vi "modify channel test.vi"() -> ()   [LabVIEW 2013, in "TEC tests.lvlib"]
uses:
  TEC tests.lvlib
  <vilib>/NI/Tag Bus Module Framework/channel/channel classification.ctl
  configuration/TEC configuration.lvclass
  configuration/TEC configuration.lvclass/TEC configuration.ctl
  <vilib>/NI/Tag Bus Module Framework/channel/TBM channel.lvclass/TBM channel.ctl
  <vilib>/NI/Tag Bus/tag/tag descriptor.lvclass/tag descriptor.ctl
  <vilib>/NI/Tag Bus Module Framework/channel/Read channel classification.vi
  <vilib>/NI/Tag Bus Module Framework/channel/Write channel classification.vi
  <vilib>/NI/Tag Bus/tag/read tag name.vi
  configuration/Write channels.vi
  <vilib>/NI/Tag Bus Module Framework/channel/TBM channel.lvclass
  <vilib>/NI/Tag Bus Module Framework/root configuration/TBM configuration.lvclass
panel:
  out "rename success":bool
  out "no err":errorcluster
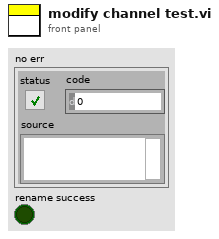
[diagram p1: front panel]
types:
  T1 = typedef "TBM channel.lvclass/channel classification.ctl" = enum16{"input data", "output data", "processing parameter", "processing result"}
  T2 = typedef "tag bus.lvlib/tag descriptor.lvclass/Data Type.ctl" = enum16{"Double", "Single", "I64", "I32", "I16", "I8", "U64", "U32", "U16", "U8", "Boolean", "String", "Array of Double", "Array of Single", "Array of I64", "Array of I32", "Array of I16", "Array of I8", "Array of U64", "Array of U32", "Array of U16", "Array of U8", "Array of Boolean", "Array of String"}
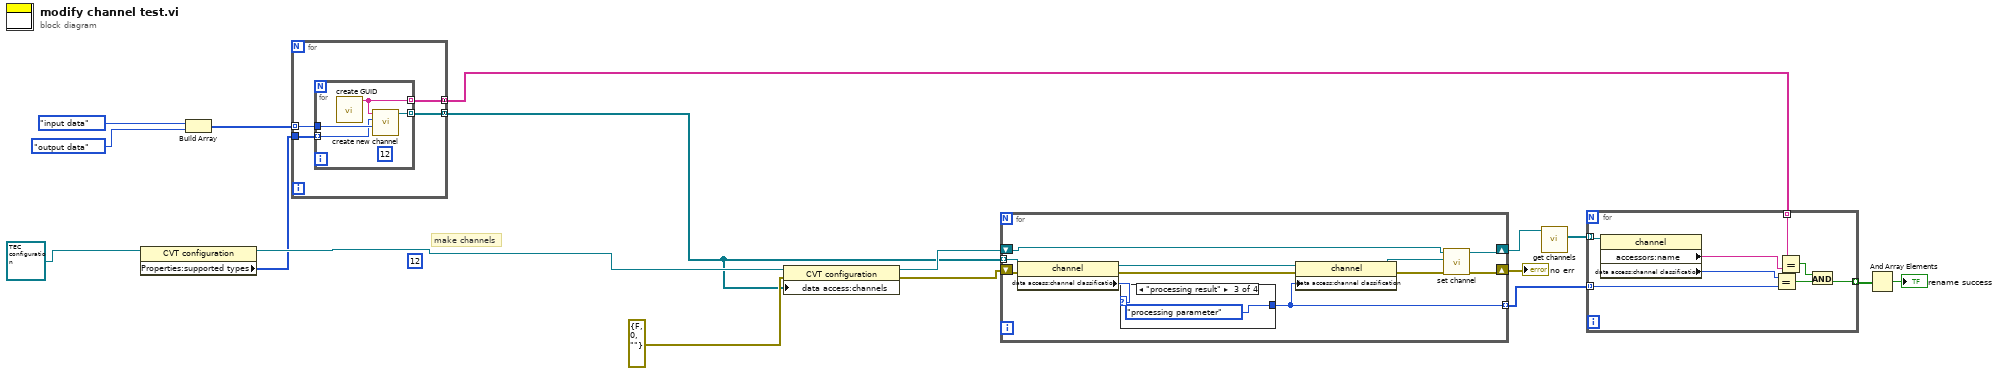
[diagram p0: block diagram]
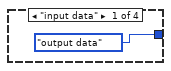
[diagram p2: hidden frame]
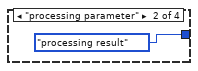
[diagram p3: hidden frame]
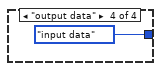
[diagram p4: hidden frame]
diagram:
  (unwired) 12
  # "make channels"
  n1 = property class="CVT configuration"(reference=refnum<class "TEC configuration.lvclass"> refnum ("tag bus configurable plugin module configuration")) -> (reference out=w14:refnum<class "TEC configuration.lvclass">, "Properties:supported types"=w13:T2[])  [unwired: 1 in, 1 out]
  n2 = Build Array(channel_classification."input data" ("channel classification"), channel_classification."output data" ("channel classification")) -> (w15:T1[])
  n3 = for {
    tunnel: w15 -> [w21] mode=indexing
    tunnel: [w19] -> w1 mode=concatenating
    tunnel: w13 -> [w20]
    tunnel: [w18] -> w6 mode=concatenating
    n4 = for {
      tunnel: w21 -> [w24]
      tunnel: [w25] -> w19 mode=indexing
      tunnel: w20 -> [w23] mode=indexing
      tunnel: [w22] -> w18 mode=indexing
      (unwired) 12
      n5 = call <vilib>:"create GUID.vi"() -> ("uuid"=w22:string)  [unwired: 11 in]
      n6 = call <vilib>:"create new channel.vi"("channel classification"=w24, "data type"=w23, "channel name"=w22) -> ("channel"=w25:refnum<class "TBM channel.lvclass">)  [unwired: 8 in]
    }
  }
  n7 = property class="CVT configuration"(reference=w14, error in=errorcluster {"status"=FALSE, "code"=0, "source"=""} ("error out"), "data access:channels"=w1) -> (reference out=w2:refnum<class "TEC configuration.lvclass">, error out=w3:errorcluster)
  n8 = for {
    shift-right: [w35] -> w12
    shift-left: w2 -> [w36]
    shift-right: [w34] -> w11
    shift-left: w3 -> [w33]
    tunnel: w1 -> [w31] mode=indexing
    tunnel: [w26] -> w7 mode=indexing
    n9 = property class="channel"(reference=w31, error in=w33) -> (reference out=w29:refnum<class "TBM channel.lvclass">, error out=w32:errorcluster, "data access:channel classification"=w27:T1)
    n10 = case shown="\"processing result\"" w27 {
      tunnel: [channel_classification."output data" ("channel classification") channel_classification."processing result" ("channel classification") channel_classification."processing parameter" ("channel classification") channel_classification."input data" ("channel classification")] -> w26
      frame "input data" {
      }
      frame "processing parameter" {
      }
      frame "processing result" {
      }
      frame "output data" {
      }
    }
    n11 = property class="channel"(reference=w29, error in=w32, "data access:channel classification"=w26) -> (reference out=w28:refnum<class "TBM channel.lvclass">, error out=w30:errorcluster)
    n12 = call "set channel.vi"("error in"=w30, "TBM channel in"=w28, "CVT configuration in"=w36) -> ("error out"=w34:errorcluster, "CVT configuration out"=w35:refnum<class "TEC configuration.lvclass">)  [unwired: 7 in]
  }
  "no err" <- w11
  n13 = call-dynamic "get channels.vi"("CVT configuration in"=w12) -> ("channels"=w10:refnum<class "TBM channel.lvclass">[])  [unwired: 9 in, 1 out]
  n14 = for {
    tunnel: w10 -> [w47] mode=indexing
    tunnel: [w46] -> w9 mode=indexing
    tunnel: w7 -> [w45] mode=indexing
    tunnel: w6 -> [w42] mode=indexing
    n15 = property class="channel"(reference=w47) -> ("accessors:name"=w43:string, "data access:channel classification"=w44:T1)  [unwired: 1 in, 2 out]
    n16 = Equal?(x=w44, y=w45) -> (x = y?=w48:bool)
    n17 = Equal?(x=w42, y=w43) -> (x = y?=w41:bool)
    n18 = And(x=w41, y=w48) -> (x .and. y?=w46:bool)
  }
  n19 = And Array Elements(Boolean array=w9) -> (logical AND=→"rename success":bool)
